vi "Read header.vi"(8 "error in (no error)":errorcluster, 11 "CoSy Config File in":refnum<class "CoSy Config File.lvclass">) -> (0 "error out":errorcluster, 2 "Config file header info":T1, 3 "CoSy Config File out":refnum<class "CoSy Config File.lvclass">)   [LabVIEW 2011, in "COSYLib.lvlib" / "CoSy Config File.lvclass"]
doc: "Reads the header information from the configuration file."
uses:
  CoSy Config File.lvclass
  Config file header info.ctl
  CoSy Config File.lvclass/CoSy Config File.ctl
  <vilib>/xml/Close Reference(Node).vi
  <vilib>/xml/NI_XML.lvlib
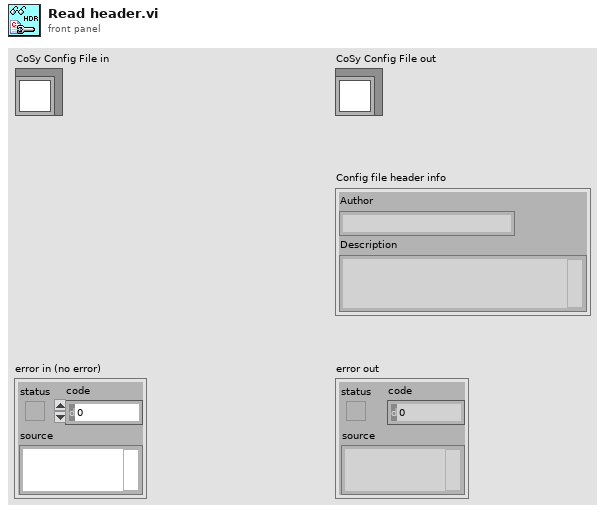
[diagram p1: front panel]
types:
  T1 = typedef "COSYLib.lvlib/CoSy Config File.lvclass/Config file header info.ctl" = cluster{"Author":string, "Description":string}
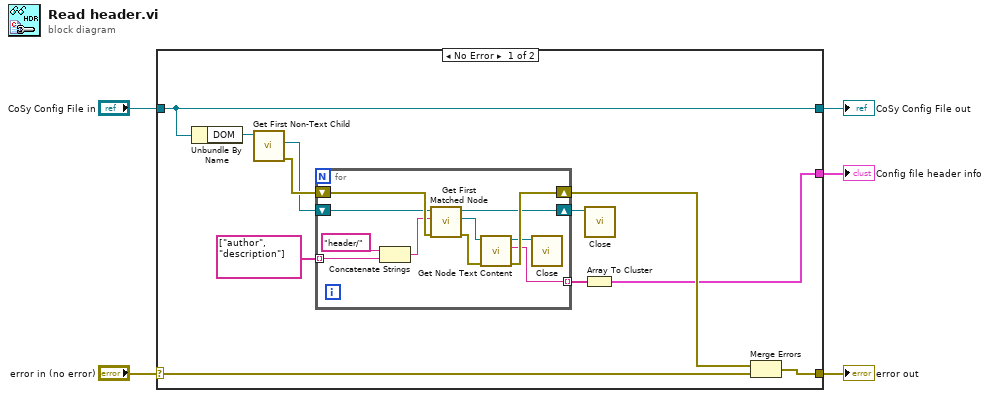
[diagram p0: block diagram]
diagram:
  n1 = case shown="No Error" "error in (no error)" {
    selector: "error in (no error)" -> [w16 w29]
    tunnel: [w14 w29] -> w4
    tunnel: [w11 w28] -> w2
    tunnel: "CoSy Config File in" -> [w11 w28]
    tunnel: [w6 _] -> w1
    frame No Error {
      n2 = Unbundle By Name(w11) -> ("DOM"=w10:refnum<k20>)
      n3 = call <vilib>:"Get First Non-Text Child.vi"("node in"=w10) -> ("error out"=w15:errorcluster, "child node"=w9:refnum<k20>)  [unwired: 7 in, 2 out]
      n4 = for {
        shift-right: [w23] -> w8
        shift-left: w9 -> [w24]
        tunnel: string[] ["author", "description"] -> [w22] mode=indexing
        tunnel: [w18] -> w7 mode=indexing
        shift-right: [w25] -> w13
        shift-left: w15 -> [w27]
        n5 = Concatenate Strings("header/" ("string"), w22) -> (w21:string)
        n6 = call <vilib>:"Get First Matched Node.vi"("error in (no error)"=w27, "XPath expression"=w21, "node in"=w24) -> ("error out"=w26:errorcluster, "node result"=w19:refnum<k20>, "node out"=w23:refnum<k20>)  [unwired: 6 in]
        n7 = call <vilib>:"Get Node Text Content.vi"("error in (no error)"=w26, "node in"=w19) -> ("error out"=w25:errorcluster, "node text"=w18:string, "node out"=w17:refnum<k20>)  [unwired: 7 in]
        n8 = call-poly <vilib>:"Close.vi"("node"=w17) -> ()  [unwired: 8 in, 1 out]
      }
      n9 = Array To Cluster(array=w7) -> (cluster=w6:cluster{"[0]":string, "[1]":string})
      n10 = call-poly <vilib>:"Close.vi"("node"=w8) -> ()  [unwired: 8 in, 1 out]
      n11 = Merge Errors(w13, w16) -> (w14:errorcluster)
    }
    frame Error {
    }
  }
  "error out" <- w4
  "CoSy Config File out" <- w2
  "Config file header info" <- w1
